vi "task2.vi"() -> ()   [LabVIEW 2021]
uses:
  <vilib>/measure/mascope.llb/Pulse Measurements 1 chan.vi
  <vilib>/Utility/file.llb/Write Delimited Spreadsheet (string).vi
  <vilib>/Utility/file.llb/Write Delimited Spreadsheet (DBL).vi
  <vilib>/measure/NI_MAPro.lvlib
panel:
  in  "reference levels":T1={"high ref level"=90.0, "mid ref level"=50.0, "low ref level"=10.0, "ref units"=1} {"ref units" items=["absolute", "percent"]; "high ref level" format="%0.2f"; "low ref level" format="%0.2f"; "mid ref level" format="%0.2f"}
  out "Duty cycle":waveform(dbl)(graph)
  out "Pulse duration":waveform(dbl)(graph)
  out "period":dbl format="%.2e"
  out "pulse duration":dbl format="%.2e"
  out "duty cycle":dbl format="%.2e"
  out "Sampling time":dbl[](graph)
  in  "Sampling rate low":dbl=250000.0
  in  "Sampling rate high":dbl=250000.0
  in  "Samples low":i32
  out "Samples low aquired":i32
  out "Waveform Graph":waveform(dbl)(graph)
  out "error out":errorcluster
  in  "Samplpes high":i32=100
  out "Period":waveform(dbl)(graph)
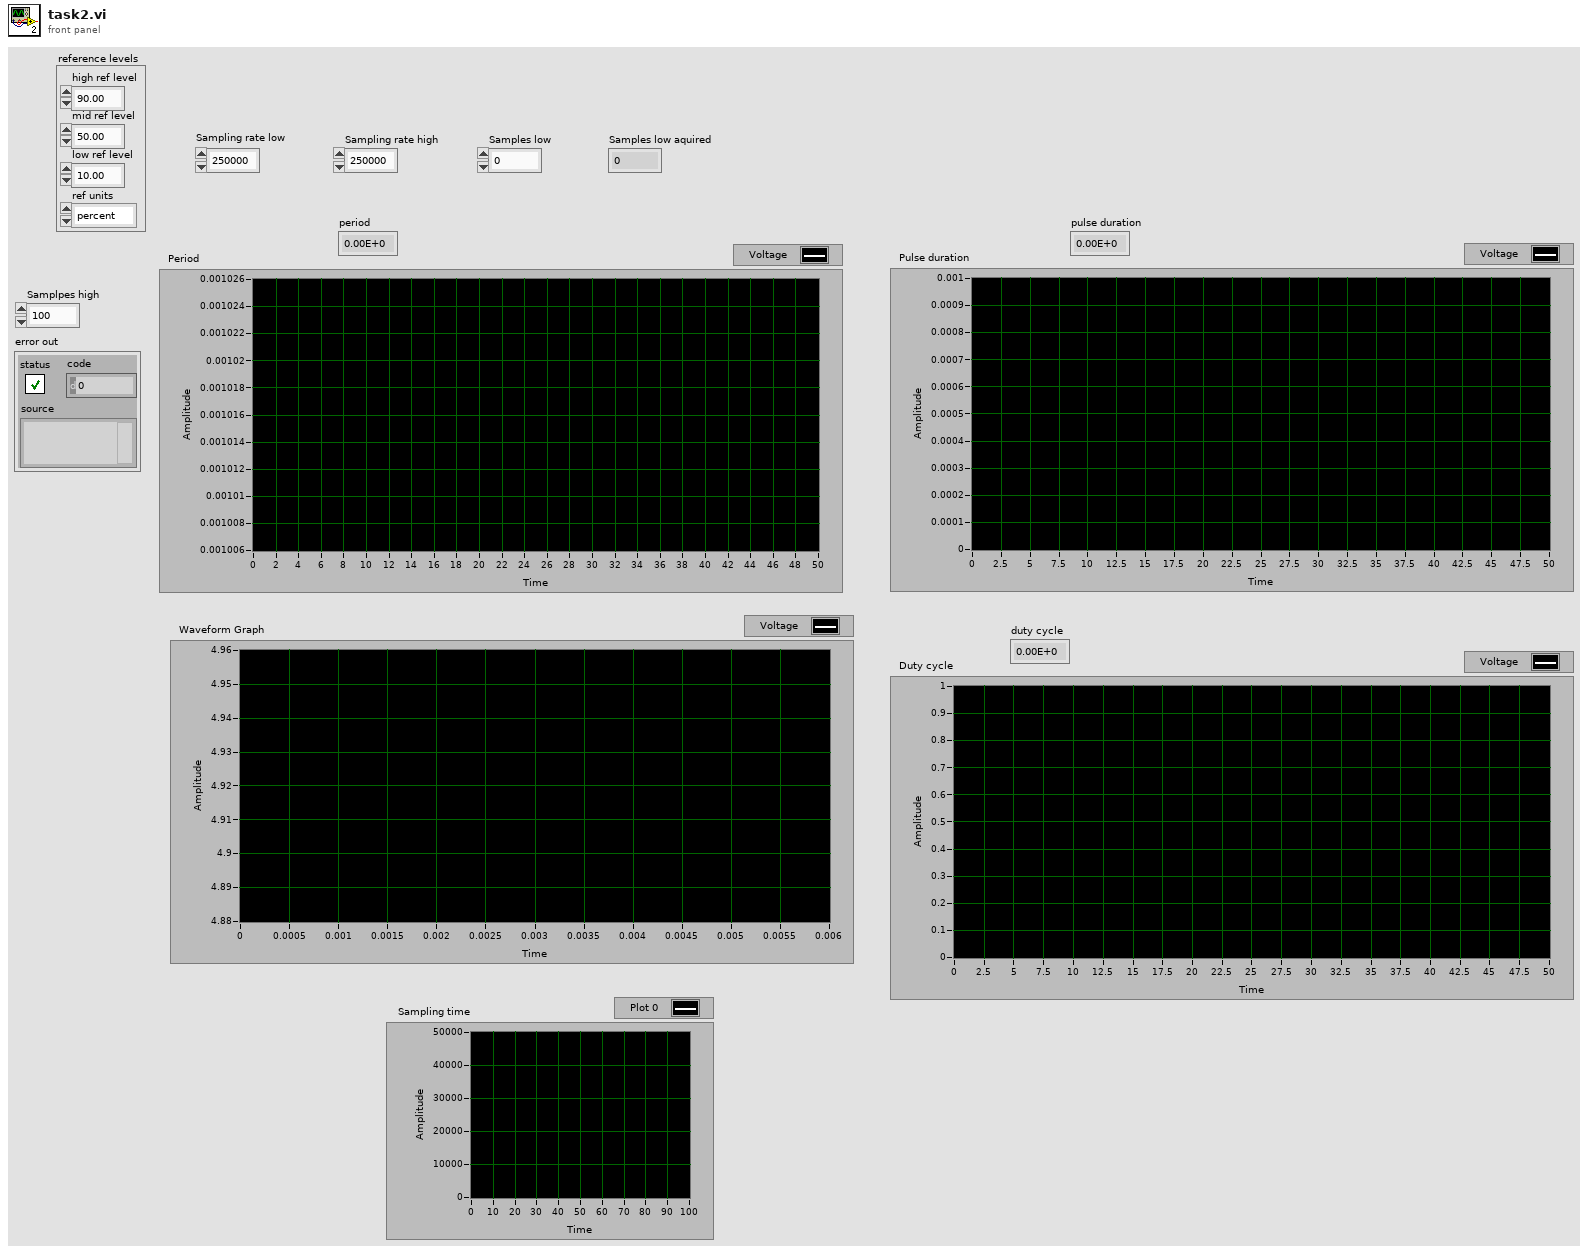
[diagram p1: front panel]
types:
  T1 = cluster{"high ref level":dbl, "mid ref level":dbl, "low ref level":dbl, "ref units":u16}
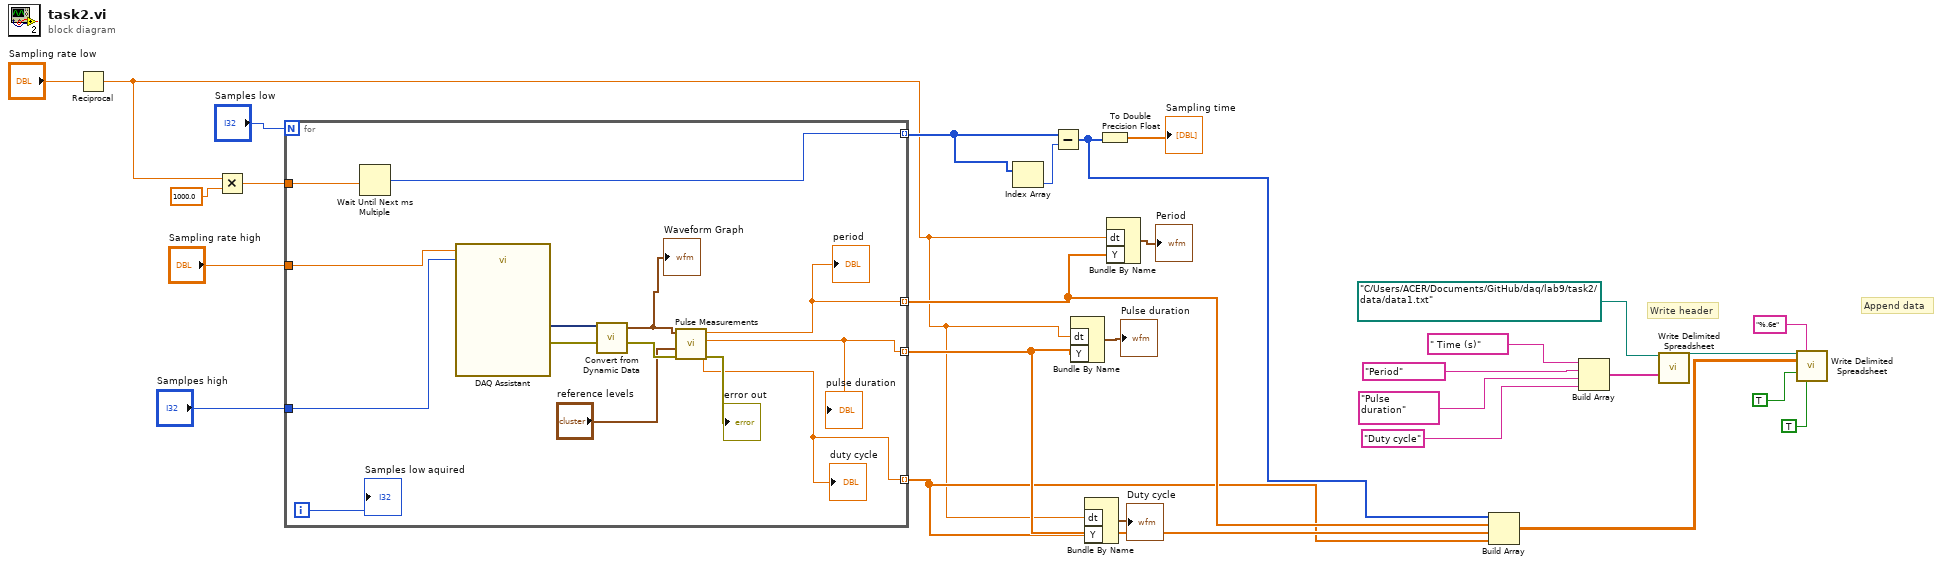
[diagram p0: block diagram]
diagram:
  # "Write header"
  # "Append data"
  n1 = Reciprocal(x="Sampling rate low") -> (1/x=w4:dbl)
  n2 = Multiply(x=w4, y=1000.0) -> (x*y=w24:dbl)
  n3 = for {
    N: "Samples low" -> [_]
    tunnel: [w31] -> w9 mode=indexing
    tunnel: "Samplpes high" -> [w38]
    tunnel: "Sampling rate high" -> [w36]
    tunnel: w24 -> [w35]
    tunnel: [w34] -> w20 mode=indexing
    tunnel: [w32] -> w6 mode=indexing
    tunnel: [w33] -> w5 mode=indexing
    i -> [w37]
    n4 = Wait Until Next ms Multiple(millisecond multiple=w35) -> (millisecond timer value=w34:u32)
    n5 = call "DAQ Assistant"("rate"=w36, "number of samples"=w38) -> ("data"=w41:dynamicdata, "error out"=w30:errorcluster)  [unwired: 15 in, 1 out]
    n6 = call "Convert from Dynamic Data"("Dynamic Data Type"=w41) -> ("Waveform"=w39:waveform(dbl))  [unwired: 3 in]
    "Waveform Graph" <- w39
    n7 = call-poly <vilib>:"Pulse Measurements.vi"("error in (no error)"=w30, "reference levels"="reference levels", "signal in"=w39) -> ("error out"=→"error out":errorcluster, "duty cycle"=w33:dbl, "pulse duration"=w32:dbl, "period"=w31:dbl)  [unwired: 4 in, 1 out]
    "duty cycle" <- w33
    "pulse duration" <- w32
    "period" <- w31
    "Samples low aquired" <- w37
  }
  n8 = Index Array(array=w20) -> (element=w21:u32)  [unwired: 1 in]
  n9 = Subtract(x=w20, y=w21) -> (x-y=w3:u32[])
  n10 = Bundle By Name("dt"=w4, "Y"=w6) -> (→"Pulse duration":waveform(dbl))  [unwired: 1 in]
  n11 = Bundle By Name("dt"=w4, "Y"=w5) -> (→"Duty cycle":waveform(dbl))  [unwired: 1 in]
  n12 = To Double Precision Float(number=w3) -> (double precision float=→"Sampling time":dbl[])
  n13 = Bundle By Name("dt"=w4, "Y"=w9) -> (→"Period":waveform(dbl))  [unwired: 1 in]
  n14 = Build Array(w3, w9, w6, w5) -> (w10:dbl[][])
  n15 = Build Array(" Time (s)" ("element"), "Period" ("format string"), "Pulse duration" ("element"), "Duty cycle" ("element")) -> (w12:string[])
  n16 = call-poly <vilib>:"Write Delimited Spreadsheet.vi"("file path (dialog if empty)"=path "C:/Users/ACER/Documents/GitHub/daq/lab9/task2/data/data1.txt", "1D data"=w12) -> ("new file path (Not A Path if cancelled)"=w17:path)  [unwired: 12 in, 1 out]
  n17 = call-poly <vilib>:"Write Delimited Spreadsheet.vi"("file path (dialog if empty)"=w17, "format (%.3f)"="%.6e", "2D data"=w10, "append to file? (new file:F)"=TRUE, "transpose? (no:F)"=TRUE) -> ()  [unwired: 9 in, 2 out]
